vi "Pots.vi"() -> ()   [LabVIEW 2013]
uses:
  <vilib>/Instr/_visa.llb/VISA Configure Serial Port (Instr).vi
panel:
  out "read buffer":string
  in  "COM:":refnum<visa-resource-name>
  out "Gauge":dbl(knob) scale=0.0..220.0
  out "Meter":dbl(knob) scale=0.0..5.0
  out "Thermometer":dbl(slide) scale=0.0..45.0
  out "Tank":dbl(slide) scale=0.0..100.0
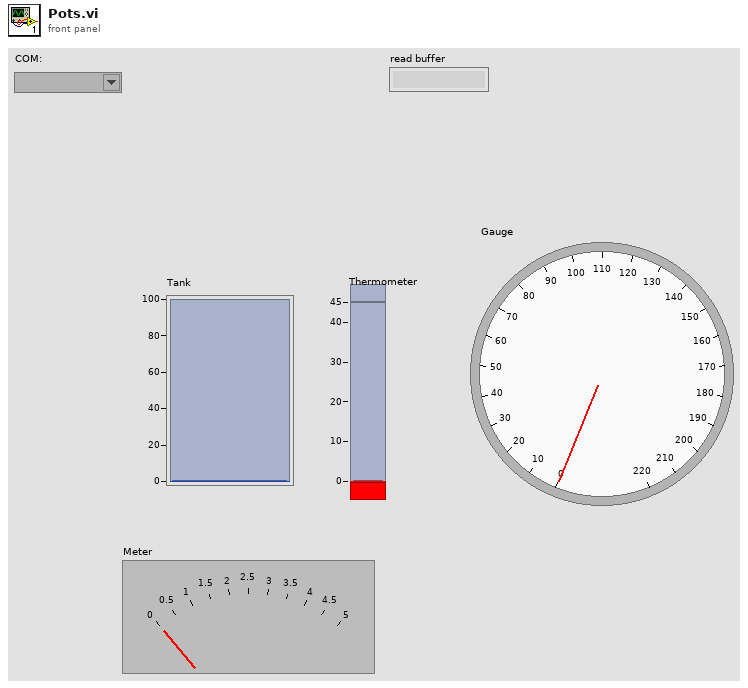
[diagram p1: front panel]
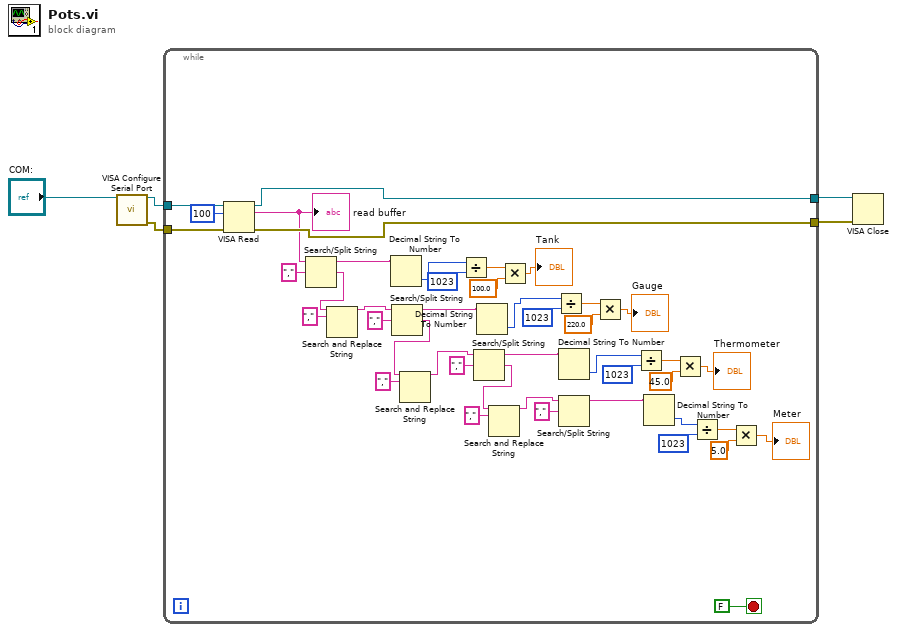
[diagram p0: block diagram]
diagram:
  n1 = call-poly "VISA Configure Serial Port"("VISA resource name"="COM:") -> ("VISA resource name out"=w4:refnum<visa-resource-name>, "error out"=w3:errorcluster)  [unwired: 13 in]
  n2 = while {
    tunnel: w4 -> [w48]
    tunnel: w3 -> [w47]
    tunnel: [w45] -> w2
    tunnel: [w44] -> w1
    stop <- FALSE stop-if-true
    n3 = VISA Read(VISA resource name=w48, byte count=u32 100, error in (no error)=w47) -> (VISA resource name out=w45:refnum<visa-resource-name>, read buffer=w43:string, error out=w44:errorcluster)  [unwired: 1 out]
    "read buffer" <- w43
    n4 = Search/Split String(string=w43, search string/char (-)=",") -> (substring before match=w20:string, match + rest of string=w14:string)  [unwired: 1 in, 1 out]
    n5 = Search and Replace String(input string=w14, search string=",") -> (result string=w12:string)  [unwired: 6 in, 3 out]
    n6 = Decimal String To Number(string=w20) -> (number=w19:i32)  [unwired: 2 in, 1 out]
    n7 = Search/Split String(string=w12, search string/char (-)=",") -> (substring before match=w15:string, match + rest of string=w9:string)  [unwired: 1 in, 1 out]
    n8 = Search and Replace String(input string=w9, search string=",") -> (result string=w8:string)  [unwired: 6 in, 3 out]
    n9 = Divide(x=w19, y=1023) -> (x/y=w35:dbl)
    n10 = Search/Split String(string=w8, search string/char (-)=",") -> (substring before match=w39:string, match + rest of string=w7:string)  [unwired: 1 in, 1 out]
    n11 = Decimal String To Number(string=w15) -> (number=w18:i32)  [unwired: 2 in, 1 out]
    n12 = Search and Replace String(input string=w7, search string=",") -> (result string=w6:string)  [unwired: 6 in, 3 out]
    n13 = Multiply(x=w35, y=100.0) -> (x*y=→"Tank":dbl)
    n14 = Divide(x=w18, y=1023) -> (x/y=w32:dbl)
    n15 = Decimal String To Number(string=w39) -> (number=w17:i32)  [unwired: 2 in, 1 out]
    n16 = Search/Split String(string=w6, search string/char (-)=",") -> (substring before match=w37:string)  [unwired: 1 in, 2 out]
    n17 = Multiply(x=w32, y=220.0) -> (x*y=→"Gauge":dbl)
    n18 = Divide(x=w17, y=1023) -> (x/y=w29:dbl)
    n19 = Decimal String To Number(string=w37) -> (number=w16:i32)  [unwired: 2 in, 1 out]
    n20 = Multiply(x=w29, y=45.0) -> (x*y=→"Thermometer":dbl)
    n21 = Divide(x=w16, y=1023) -> (x/y=w26:dbl)
    n22 = Multiply(x=w26, y=5.0) -> (x*y=→"Meter":dbl)
  }
  n23 = VISA Close(VISA resource name=w2, error in (no error)=w1) -> ()  [unwired: 1 out]
